vi "LV2010plus_PostInstall.vi"(8 "error in":errorcluster, 11 "installed files":path[](array[path])) -> (0 "error out":errorcluster)   [LabVIEW 2010]
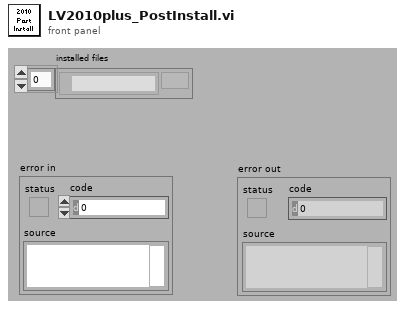
[diagram p1: front panel]
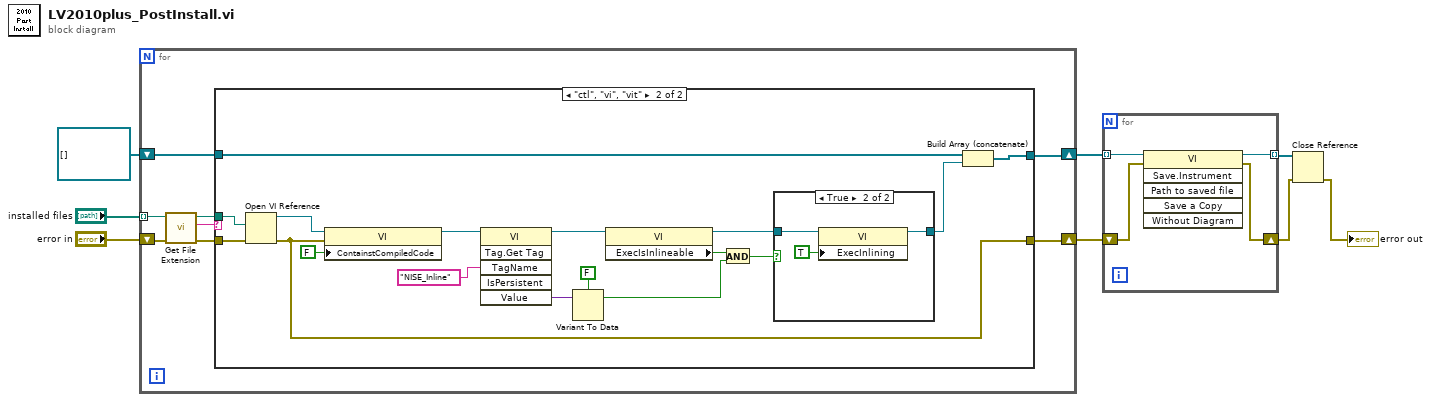
[diagram p0: block diagram]
diagram:
  n1 = for {
    tunnel: "installed files" -> [w16] mode=indexing
    shift-right: [w11] -> w4
    shift-left: "error in" -> [w15]
    shift-right: [w10] -> w5
    shift-left: refnum<vi>[] [] -> [w9]
    n2 = call <vilib>:"Get File Extension.vi"("error in (no error)"=w15, "file"=w16) -> ("error out"=w12:errorcluster, "lowercase file extension"=w14:string, "dup file"=w13:path)  [unwired: 6 in, 1 out]
    n3 = case shown="\"ctl\", \"vi\", \"vit\"" w14 {
      tunnel: w13 -> [_ w35]
      tunnel: w12 -> [w18 w34]
      tunnel: [w18 w24] -> w11
      tunnel: [w17 w26] -> w10
      tunnel: w9 -> [w17 w25]
      frame Default {
      }
      frame "ctl", "vi", "vit" {
        n4 = Open VI Reference(vi path=w35, error in (no error)=w34) -> (vi reference=w33:refnum<vi>, error out=w24:errorcluster)  [unwired: 4 in]
        n5 = property class="VI"(reference=w33, error in=w24, "ContainstCompiledCode"=FALSE ("Contains Compiled Code")) -> (reference out=w31:refnum<vi>)  [unwired: 1 out]
        n6 = invoke class="VI" method="Tag.Get Tag"(reference=w31, "TagName"="NISE_Inline" ("Tag Name")) -> (reference out=w23:refnum<vi>, "Value"=w29:variant)  [unwired: 4 in, 4 out]
        n7 = Variant To Data(Variant=w29, type=FALSE) -> (data=w20:bool)  [unwired: 1 in, 1 out]
        n8 = property class="VI"(reference=w23) -> (reference out=w22:refnum<vi>, "ExecIsInlineable"=w21:bool)  [unwired: 1 in, 1 out]
        n9 = And(x=w21, y=w20) -> (x .and. y?=w19:bool)
        n10 = case shown="True" w19 {
          tunnel: w22 -> [w36 w39]
          tunnel: [w36 w37] -> w27
          frame False {
          }
          frame True {
            n11 = property class="VI"(reference=w39, "ExecInlining"=TRUE ("Execution:Inline SubVI")) -> (reference out=w37:refnum<vi>)  [unwired: 1 in, 1 out]
          }
        }
        n12 = Build Array (concatenate)(w25, w27) -> (w26:refnum<vi>[])
      }
    }
  }
  n13 = for {
    tunnel: w5 -> [w43] mode=indexing
    shift-right: [w41] -> w2
    shift-left: w4 -> [w42]
    tunnel: [w40] -> w3 mode=indexing
    n14 = invoke class="VI" method="Save.Instrument"(reference=w43, error in=w42) -> (reference out=w40:refnum<vi>, error out=w41:errorcluster)  [unwired: 4 in, 4 out]
  }
  n15 = Close Reference(reference=w3, error in (no error)=w2) -> (error out=→"error out":errorcluster)
